vi "Example - Authenticate using WAMP-CRA and PBKDF2-SHA-256.vi"() -> ()   [LabVIEW 2020, in "wamplv.lvlib"]
uses:
  wamplv.lvlib
  Private/PBKDF2 serialisation method.ctl
  WAMP Client/WAMP Client.lvclass/WAMP Client.ctl
  WAMP Client/API/WAMP/Publish.vi/5e405bcd-0c6d-46be-a87b-06ec174a83c2.vi
  WAMP Client/API/WAMP/Publish (async).vi
  WAMP Client/Private/SubVIs/Raise Internal Message.vi
  WAMP Client/API/WAMP/Publish (async).vi/56cb05c7-ccfa-42e5-a428-2bd237dbc257.vi
  WAMP Client/Private/Authentication/Add WAMP-CRA authenticator.vi
  <vilib>/Utility/error.llb/Error Cluster From Error Code.vi
  WAMP Client/WAMP Client.lvclass
panel:
  in  "PBKDF2 serialisation method":T1
  in  "WAMP-CRA secret (e.g. password)":string="secret"
  in  "Authorisation ID (e.g.username)":string="username"
  in  "Arguments":string
  in  "Topic URI":string="test.topic"
  in  "Realm":string="private_realm"
  in  "Router URL":string="ws://localhost:8080/"
  # "Example: uthentication with WAMP-CRA and PBKDF2-SHA-256, and publish"
  # "The WAMPs pecification does not specify how the PBKDF2 hash should be serialised\nto a string. So the wamplv library allows you to choose beteween the possible options."
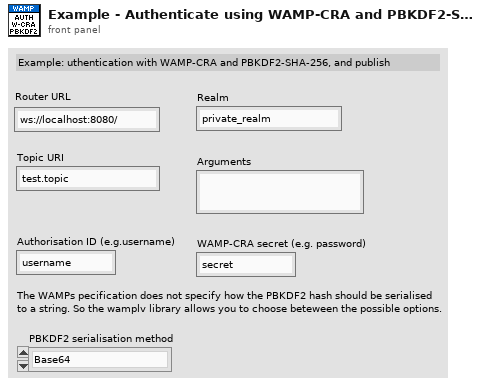
[diagram p1: front panel]
types:
  T1 = typedef "wamplv.lvlib/PBKDF2 serialisation method.ctl" = enum8{"Base64", "Hex string, lower case", "Hex string, upper case", "Direct to string cast"}
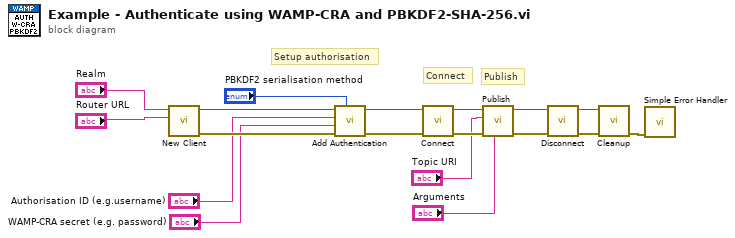
[diagram p0: block diagram]
diagram:
  # "Setup authorisation"
  # "Publish"
  # "Connect"
  n1 = call "New Client.vi"("Address"="Router URL", "Realm"="Realm") -> ("error out"=w6:errorcluster, "WAMP client out"=w7:refnum<class "WAMP Client.lvclass">)  [unwired: 8 in]
  n2 = call-poly "Add Authentication.vi"("PBKDF2 hash type"="PBKDF2 serialisation method", "error in (no error)"=w6, "Secret"="WAMP-CRA secret (e.g. password)", "Authentication ID"="Authorisation ID (e.g.username)", "WAMP Client in"=w7) -> ("error out"=w2:errorcluster, "WAMP Client out"=w3:refnum<class "WAMP Client.lvclass">)  [unwired: 5 in]
  n3 = call "Connect.vi"("error in"=w2, "WAMP Client in"=w3) -> ("error out"=w11:errorcluster, "WAMP Client out"=w13:refnum<class "WAMP Client.lvclass">)  [unwired: 8 in]
  n4 = call "Publish.vi"("Arguments"="Arguments", "Error in"=w11, "Topic"="Topic URI", "WAMP Client in"=w13) -> ("Error out"=w10:errorcluster, "WAMP Client out"=w12:refnum<class "WAMP Client.lvclass">)  [unwired: 5 in, 1 out]
  n5 = call-dynamic "Disconnect.vi"("error in"=w10, "WAMP Client in"=w12) -> ("error out"=w14:errorcluster, "WAMP Client out"=w16:refnum<class "WAMP Client.lvclass">)  [unwired: 8 in]
  n6 = call-dynamic "Cleanup.vi"("error in"=w14, "WAMP Client in"=w16) -> ("error out"=w15:errorcluster)  [unwired: 8 in, 1 out]
  n7 = call <vilib>:"Simple Error Handler.vi"("error in (no error)"=w15) -> ()  [unwired: 4 in, 5 out]
